vi "OFDM_SymbolMaping.vi"(8 "error in (no error)":errorcluster, 10 "Modulation type":enum16{"QPSK(4QAM)", "64QAM", "16QAM", "BPSK"}(ring), 11 "input bit stream":i8[](array[numeric])) -> (0 "error out":errorcluster, 3 "symbols":cdb[](array[numeric]))   [LabVIEW 2018]
uses:
  <vilib>/addons/Modulation/Digital/General/MT Map Bits to QAM Symbols.vi
  <vilib>/addons/Modulation/Digital/General/MT Map Bits to PSK Symbols.vi
  <vilib>/addons/Modulation/niDMT.lvlib
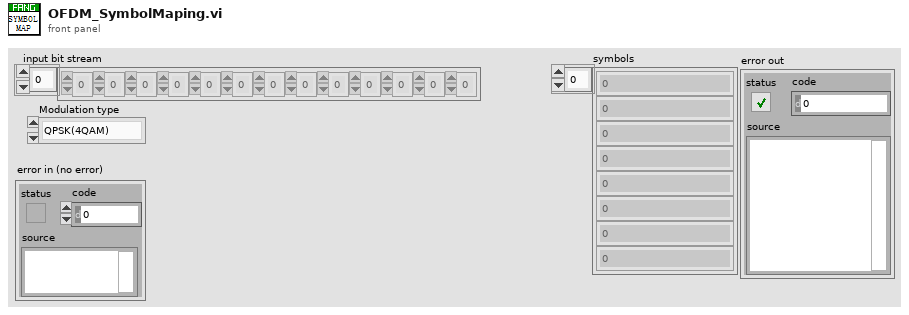
[diagram p1: front panel]
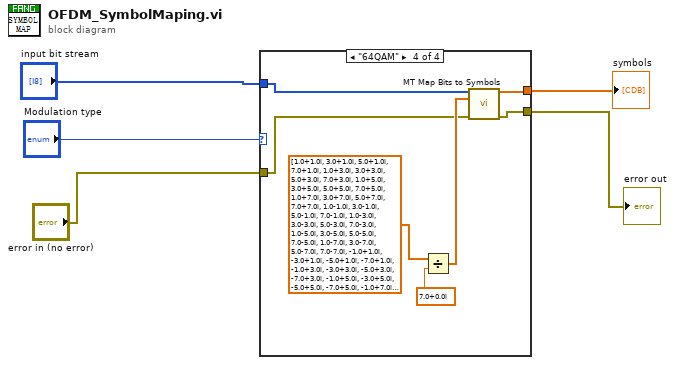
[diagram p0: block diagram]
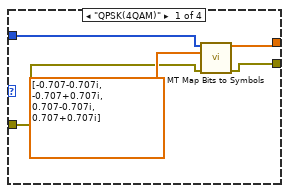
[diagram p2: hidden frame]
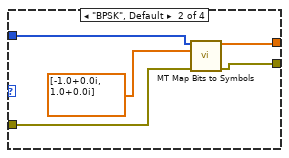
[diagram p3: hidden frame]
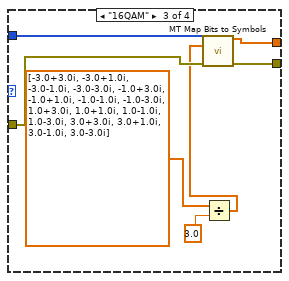
[diagram p4: hidden frame]
diagram:
  n1 = case shown="\"64QAM\"" "Modulation type" {
    tunnel: [w10 w11 w20 w23] -> w2
    tunnel: "error in (no error)" -> [w7 w13 w22 w25]
    tunnel: "input bit stream" -> [w9 w15 w21 w26]
    tunnel: [w6 w12 w19 w24] -> w1
    frame "QPSK(4QAM)" {
      n2 = call-poly <vilib>:"MT Map Bits to Symbols.vi"("input bit stream"=w9, "symbol map"=cdb[] [-0.707-0.707i, -0.707+0.707i, 0.707-0.707i, 0.707+0.707i], "error in (no error)"=w7) -> ("symbols"=w10:cdb[], "error out"=w6:errorcluster)  [unwired: 11 in]
    }
    frame "BPSK", Default {
      n3 = call-poly <vilib>:"MT Map Bits to Symbols.vi"("input bit stream"=w15, "symbol map"=cdb[] [-1.0+0.0i, 1.0+0.0i], "error in (no error)"=w13) -> ("symbols"=w11:cdb[], "error out"=w12:errorcluster)  [unwired: 11 in]
    }
    frame "16QAM" {
      n4 = Divide(x=cdb[] [-3.0+3.0i, -3.0+1.0i, -3.0-1.0i, -3.0-3.0i, -1.0+3.0i, -1.0+1.0i, -1.0-1.0i, -1.0-3.0i, 1.0+3.0i, 1.0+1.0i, 1.0-1.0i, 1.0-3.0i, 3.0+3.0i, 3.0+1.0i, 3.0-1.0i, 3.0-3.0i] ("symbol map"), y=3.0) -> (x/y=w16:cdb[])
      n5 = call-poly <vilib>:"MT Map Bits to Symbols.vi"("input bit stream"=w21, "symbol map"=w16, "error in (no error)"=w22) -> ("symbols"=w20:cdb[], "error out"=w19:errorcluster)  [unwired: 11 in]
    }
    frame "64QAM" {
      n6 = Divide(x=cdb[] [1.0+1.0i, 3.0+1.0i, 5.0+1.0i, 7.0+1.0i, 1.0+3.0i, 3.0+3.0i, 5.0+3.0i, 7.0+3.0i, 1.0+5.0i, 3.0+5.0i, 5.0+5.0i, 7.0+5.0i, 1.0+7.0i, 3.0+7.0i, 5.0+7.0i, 7.0+7.0i, 1.0-1.0i, 3.0-1.0i, 5.0-1.0i, 7.0-1.0i, 1.0-3.0i, 3.0-3.0i, 5.0-3.0i, 7.0-3.0i, 1.0-5.0i, 3.0-5.0i, 5.0-5.0i, 7.0-5.0i, 1.0-7.0i, 3.0-7.0i, 5.0-7.0i, 7.0-7.0i, -1.0+1.0i, -3.0+1.0i, -5.0+1.0i, -7.0+1.0i, -1.0+3.0i, -3.0+3.0i, -5.0+3.0i, -7.0+3.0i, -1.0+5.0i, -3.0+5.0i, -5.0+5.0i, -7.0+5.0i, -1.0+7.0i, -3.0+7.0i, -5.0+7.0i, -7.0+7.0i, -1.0-1.0i, -3.0-1.0i, -5.0-1.0i, -7.0-1.0i, -1.0-3.0i, -3.0-3.0i, -5.0-3.0i, -7.0-3.0i, -1.0-5.0i, -3.0-5.0i, -5.0-5.0i, -7.0-5.0i, -1.0-7.0i, -3.0-7.0i, -5.0-7.0i, -7.0-7.0i] ("appended array"), y=cdb 7.0+0.0i) -> (x/y=w28:cdb[])
      n7 = call-poly <vilib>:"MT Map Bits to Symbols.vi"("input bit stream"=w26, "symbol map"=w28, "error in (no error)"=w25) -> ("symbols"=w23:cdb[], "error out"=w24:errorcluster)  [unwired: 11 in]
    }
  }
  "symbols" <- w2
  "error out" <- w1
